vi "FGV_DOCK_batch_ID_buffer.vi"(7 "options":T1, 8 "error_in":errorcluster, 10 "BATCH_ID":string, 11 "BATCH_CODE":string) -> (0 "error_out":errorcluster, 2 "Batch exists?":bool, 3 "ID_out":string)   [LabVIEW 2019]
uses:
  FGV_DOCK_batch_ID_buffer.ctl
  DOCK_batch_ID_buffer_all_info.ctl
  SQL_connection/FGV_DOCK_SQL_connection.ctl
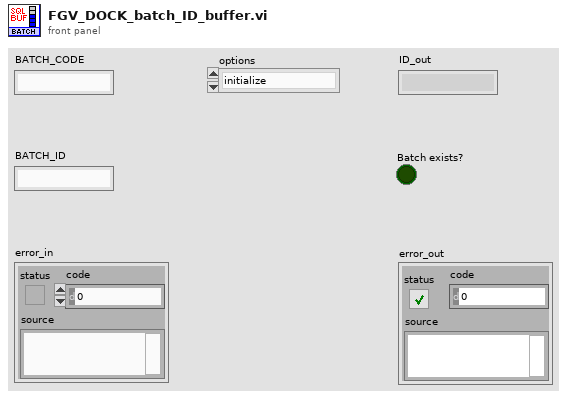
[diagram p1: front panel]
types:
  T1 = typedef "FGV_DOCK_batch_ID_buffer.ctl" = enum16{"initialize", "buffer_batch_ID", "get_ID_for_batch"}
  T2 = typedef "DOCK_batch_ID_buffer_all_info.ctl" = cluster{"BATCH_CODE_and_ID":string[][], "BATCH_CODE_and_ID_buffer_pos":i32, "BATCH_CODE_and_ID_buffer_max_size":i32}
  T3 = typedef "FGV_DOCK_SQL_connection.ctl" = enum16{"initialize", "connect", "read_tables", "read_columns", "SELECT", "INSERT", "UPDATE", "DELETE", "EXEC + headers", "EXEC", "TRANSACTION", "connection_active?", "disconnect"}
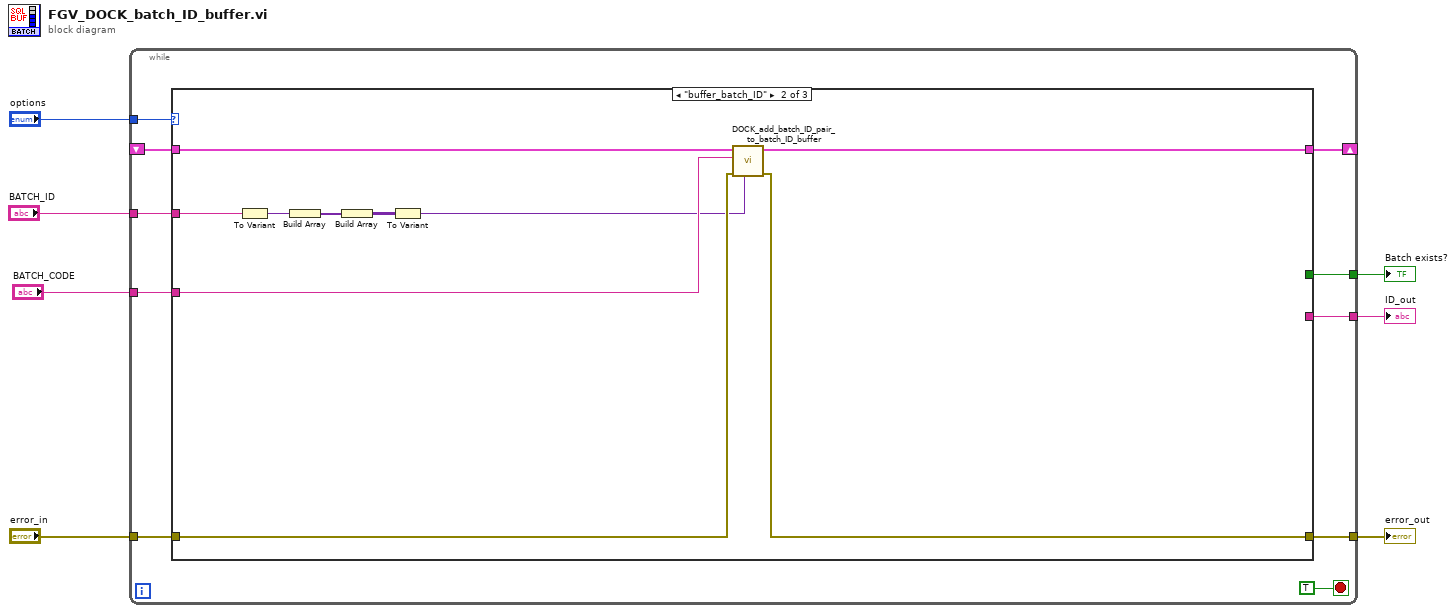
[diagram p0: block diagram]
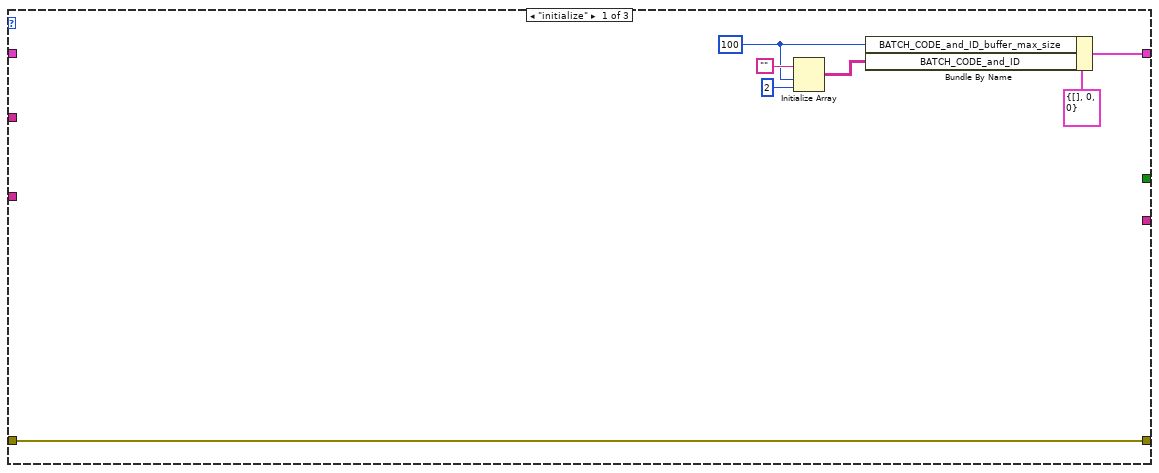
[diagram p2: hidden frame]
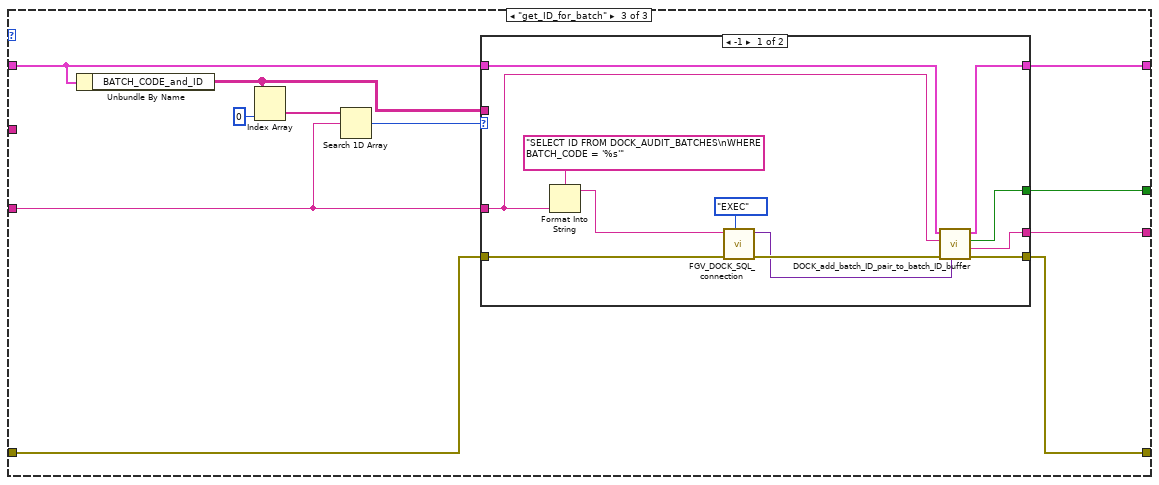
[diagram p3: hidden frame]
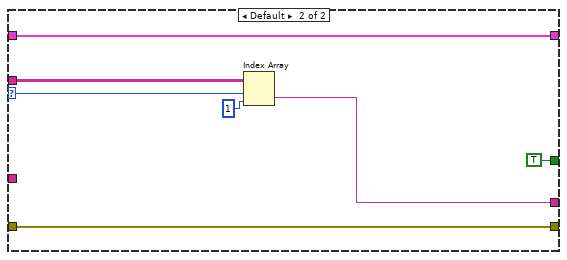
[diagram p4: hidden frame]
diagram:
  n1 = while {
    tunnel: "options" -> [w16]
    tunnel: [w15] -> w7
    tunnel: "error_in" -> [w14]
    shift-right: [w13] -> _
    shift-left: _ -> [w12]
    tunnel: "BATCH_CODE" -> [w11]
    tunnel: [w10] -> w3
    tunnel: [w9] -> w2
    tunnel: "BATCH_ID" -> [w8]
    stop <- TRUE stop-if-true
    n2 = case shown="\"buffer_batch_ID\"" w16 {
      tunnel: [w24 w31 w38] -> w15
      tunnel: w14 -> [w24 w29 w39]
      tunnel: [w18 w32 w36] -> w13
      tunnel: w12 -> [_ w33 w37]
      tunnel: w11 -> [_ w34 w40]
      tunnel: [_ _ w41] -> w10
      tunnel: [_ _ w35] -> w9
      tunnel: w8 -> [_ w30 _]
      frame "initialize" {
        w20 = 100 ("dimension size")
        n3 = Initialize Array("", w20, 2 ("dimension size")) -> (w23:string[][])
        n4 = Bundle By Name(cluster=T2 {"BATCH_CODE_and_ID"=[], "BATCH_CODE_and_ID_buffer_pos"=0, "BATCH_CODE_and_ID_buffer_max_size"=0} ("SQL_pinion_ID_buffer_all_info"), "BATCH_CODE_and_ID_buffer_max_size"=w20, "BATCH_CODE_and_ID"=w23) -> (w18:T2)
      }
      frame "buffer_batch_ID" {
        n5 = To Variant(anything=w30) -> (Variant=w28:variant)
        n6 = Build Array(w28) -> (w27:variant[])
        n7 = Build Array(w27) -> (w26:variant[][])
        n8 = To Variant(anything=w26) -> (Variant=w25:variant)
        n9 = call "DOCK_add_batch_ID_pair_to_batch_ID_buffer.vi"("SQL_result"=w25, "error_in"=w29, "BATCH_CODE"=w34, "SQL_pinion_ID_buffer_all_info_in"=w33) -> ("error_out"=w31:errorcluster, "SQL_pinion_ID_buffer_all_info_out"=w32:T2)  [unwired: 4 in, 2 out]
      }
      frame "get_ID_for_batch" {
        n10 = Unbundle By Name(w37) -> ("BATCH_CODE_and_ID"=w42:string[][])
        n11 = Index Array(array=w42, index (col)=0 ("disabled index (col)")) -> (element=w44:string[])  [unwired: 1 in]
        n12 = Search 1D Array(1D array=w44, element=w40) -> (index of element=w43:i32)  [unwired: 1 in]
        n13 = case shown="-1" w43 {
          selector: w43 -> [_ w64]
          tunnel: w42 -> [_ w63]
          tunnel: [w52 w61] -> w41
          tunnel: w40 -> [w53 _]
          tunnel: w39 -> [w50 w60]
          tunnel: [w56 w60] -> w38
          tunnel: w37 -> [w55 w59]
          tunnel: [w54 w59] -> w36
          tunnel: [w51 TRUE ("Part exists?")] -> w35
          frame -1 {
            n14 = Format Into String(format string="SELECT ID FROM DOCK_AUDIT_BATCHES\nWHERE BATCH_CODE = '%s'", w53) -> (resulting string=w47:string)  [unwired: 2 in, 1 out]
            n15 = call "FGV_DOCK_SQL_connection.vi"("options"=FGV_DOCK_SQL_connection."EXEC", "error_in"=w50, "SQL_statement"=w47) -> ("error_out"=w49:errorcluster, "SQL_result"=w46:variant)  [unwired: 4 in, 3 out]
            n16 = call "DOCK_add_batch_ID_pair_to_batch_ID_buffer.vi"("SQL_result"=w46, "error_in"=w49, "BATCH_CODE"=w53, "SQL_pinion_ID_buffer_all_info_in"=w55) -> ("error_out"=w56:errorcluster, "BATCH_ID_out"=w52:string, "Batch exists?"=w51:bool, "SQL_pinion_ID_buffer_all_info_out"=w54:T2)  [unwired: 4 in]
          }
          frame Default {
            n17 = Index Array(array=w63, index (row)=w64, index (col)=1 ("disabled index (col)")) -> (element=w61:string)
          }
        }
      }
    }
  }
  "error_out" <- w7
  "ID_out" <- w3
  "Batch exists?" <- w2
